vi "Affichage calculs maths.vi"(11 "Calculs maths":dbl[](array[numeric])) -> ()   [LabVIEW 2015]
panel:
  out "Résidus ajust. exp":dbl caption="Moyenne 6"
  out "Offset ajust. exp":dbl caption="Variance ="
  out "Atténuation ajust. exp":dbl caption="Ecart type ="
  out "Amplitude ajust. exp":dbl caption="Max ="
  out "R²":dbl caption="Min ="
  out "Résidus just. lin.":dbl caption="Moyenne ="
  out "Offset ajust. lin.":dbl
  out "Pente ajust. lin.":dbl
  out "Intégrale":dbl caption="Moyenne 6"
  out "Variance":dbl caption="Variance ="
  out "Ecart type":dbl caption="Ecart type ="
  out "Max":dbl caption="Max ="
  out "Min":dbl caption="Min ="
  out "Moyenne":dbl caption="Moyenne ="
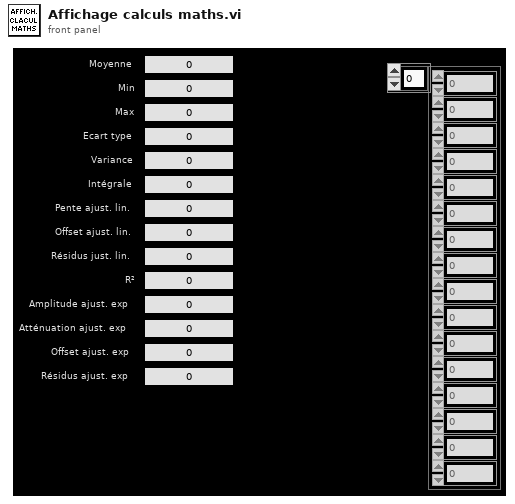
[diagram p1: front panel]
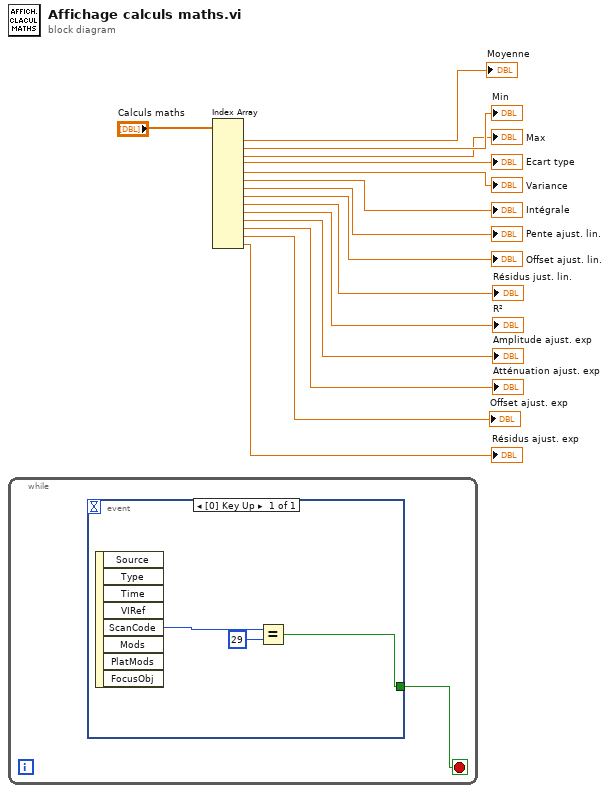
[diagram p0: block diagram]
diagram:
  n1 = while {
    stop <- w16 stop-if-true
    n2 = event shown="[0] Key Up" {
      selector: _ -> [_]
      dyn-events: _ -> [_]
      timeout: _ -> [_]
      tunnel: [w17] -> w16
      event Key Up {
        n3 = event-data() -> ("ScanCode"=w19:i16)  [unwired: 1 in, 7 out]
        n4 = Equal?(x=w19, y=i16 29) -> (x = y?=w17:bool)
      }
    }
  }
  n5 = Index Array(array="Calculs maths") -> (element #1=→"Moyenne":dbl, element #2=→"Min":dbl, element #3=→"Max":dbl, element #4=→"Ecart type":dbl, element #5=→"Variance":dbl, element #6=→"Intégrale":dbl, element #7=→"Pente ajust. lin.":dbl, element #8=→"Offset ajust. lin.":dbl, element #9=→"Résidus just. lin.":dbl, element #10=→"R²":dbl, element #11=→"Amplitude ajust. exp":dbl, element #12=→"Atténuation ajust. exp":dbl, element #13=→"Offset ajust. exp":dbl, element #14=→"Résidus ajust. exp":dbl)  [unwired: 14 in]
